vi "polish.vi"(0 "VI Ref In":refnum<vi>, 1 "VI Path":path, 11 "error in":errorcluster, 12 "Ctrl Sequences":string[](array[string])) -> (4 "VI Ref Out":refnum<vi>, 15 "error out":errorcluster)   [LabVIEW 2018]
uses:
  Common/VI Scripting/VI/Connector/Connector.lvlib
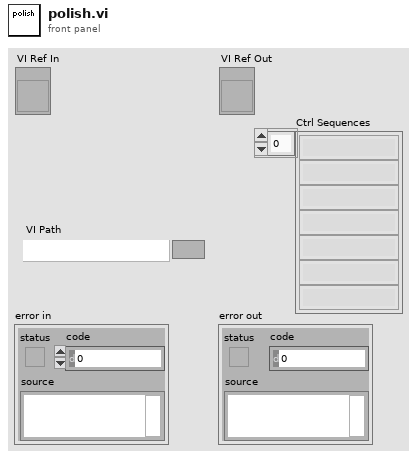
[diagram p1: front panel]
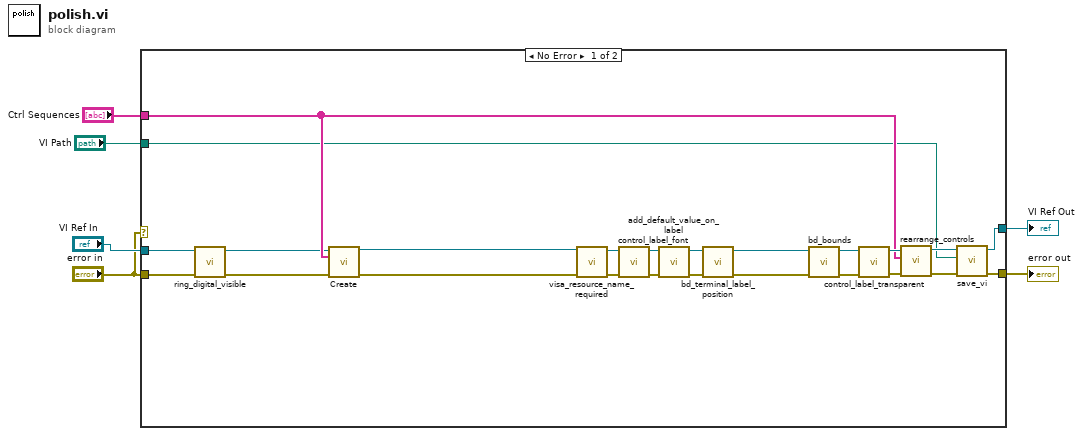
[diagram p0: block diagram]
diagram:
  n1 = case shown="No Error" "error in" {
    selector: "error in" -> [_ w32]
    tunnel: "error in" -> [w30 _]
    tunnel: "VI Ref In" -> [w29 w31]
    tunnel: [w28 w32] -> w5
    tunnel: [w27 w31] -> w4
    tunnel: "VI Path" -> [w21 _]
    tunnel: "Ctrl Sequences" -> [w22 _]
    frame No Error {
      n2 = call "ring_digital_visible.vi"("error in (no error)"=w30, "VI Ref In"=w29) -> ("error out"=w7:errorcluster, "VI Ref Out"=w8:refnum<vi>)  [unwired: 8 out]
      n3 = call "Create.vi"("vi reference"=w8, "Ctrl Sequences"=w22, "error in (no error)"=w7) -> ("vi reference out"=w16:refnum<vi>, "error out"=w9:errorcluster)  [unwired: 11 out]
      n4 = call "visa_resource_name_required.vi"("error in (no error)"=w9, "VI Ref"=w16) -> ("error out"=w17:errorcluster, "VI Ref Out"=w18:refnum<vi>)  [unwired: 8 out]
      n5 = call "control_label_font.vi"("error in (no error)"=w17, "VI Ref In"=w18) -> ("error out"=w12:errorcluster, "VI Ref Out"=w13:refnum<vi>)  [unwired: 8 out]
      n6 = call "add_default_value_on_label.vi"("error in (no error)"=w12, "VI Ref In"=w13) -> ("error out"=w19:errorcluster, "VI Ref Out"=w20:refnum<vi>)  [unwired: 8 out]
      n7 = call "bd_terminal_label_position.vi"("error in (no error)"=w19, "VI Ref In"=w20) -> ("error out"=w10:errorcluster, "VI Ref Out"=w11:refnum<vi>)  [unwired: 8 out]
      n8 = call "bd_bounds.vi"("error in (no error)"=w10, "VI Refnum"=w11) -> ("error out"=w14:errorcluster, "VI Refnum Out"=w15:refnum<vi>)  [unwired: 8 out]
      n9 = call "control_label_transparent.vi"("error in (no error)"=w14, "VI Ref In"=w15) -> ("error out"=w25:errorcluster, "VI Ref Out"=w26:refnum<vi>)  [unwired: 8 out]
      n10 = call "rearrange_controls.vi"("error in"=w25, "Ctrl Sequences"=w22, "vi reference in"=w26) -> ("error out"=w24:errorcluster, "vi reference out"=w23:refnum<vi>)  [unwired: 7 out]
      n11 = call "save_vi.vi"("error in (no error)"=w24, "VI Path"=w21, "vi reference"=w23) -> ("error out"=w28:errorcluster, "vi reference out"=w27:refnum<vi>)  [unwired: 7 out]
    }
    frame Error {
    }
  }
  "error out" <- w5
  "VI Ref Out" <- w4
